vi "Wait.vi"(8 "error in (no error)":errorcluster, 10 "wait (0ms)":u32) -> (0 "error out":errorcluster)   [LabVIEW 2020, in "Wait.lvlib"]
uses:
  Wait.lvlib
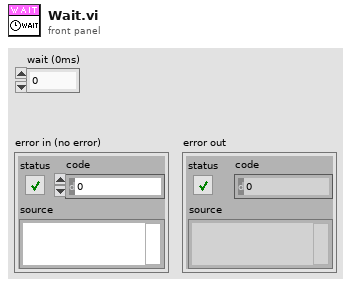
[diagram p1: front panel]
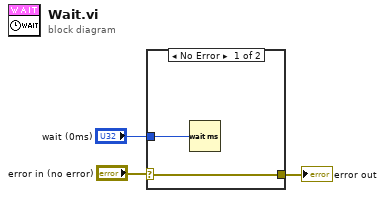
[diagram p0: block diagram]
diagram:
  n1 = case shown="No Error" "error in (no error)" {
    selector: "error in (no error)" -> [w4 w6]
    tunnel: "wait (0ms)" -> [w5 _]
    tunnel: [w4 w6] -> w1
    frame No Error {
      n2 = Wait (ms)(milliseconds to wait=w5) -> ()  [unwired: 1 out]
    }
    frame Error {
    }
  }
  "error out" <- w1
